vi "rate (SubVI).vi"(9 "new element/subarray":i32=3, 10 "direction":i32, 11 "Array in":i32[](array[numeric])) -> (3 "Array out":i32[](array[numeric]))   [LabVIEW 2020]
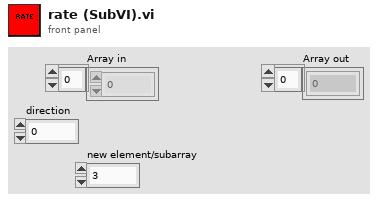
[diagram p1: front panel]
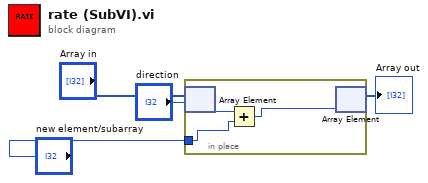
[diagram p0: block diagram]
diagram:
  n1 = in-place {
    in-place-border: "new element/subarray" -> [w5]
    n2 = in-place-array #1("Array in", "direction") -> (w7:i32)
    n3 = Add(x=w7, y=w5) -> (x+y=w6:i32)
    n4 = in-place-array #1(w6) -> (→"Array out":i32[])  [unwired: 1 out]
  }
